vi "LVImplmentation.vi"() -> ()   [LabVIEW 2017]
panel:
  out "Time":dbl
  out "Total":i32
  in  "Multiplier 2":i32
  out "Array 2":i32[](array[numeric])
  out "sum 2":i32
  out "sum":i32
  out "Array":i32[](array[numeric])
  in  "StopThrehold":i32
  in  "Multiplier":i32
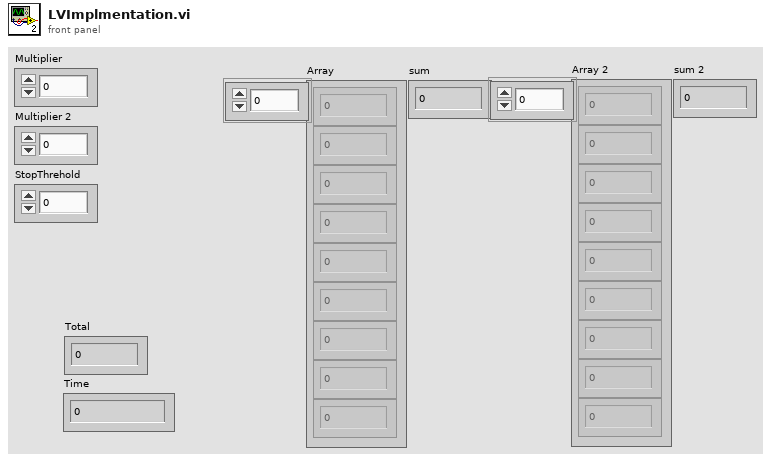
[diagram p1: front panel]
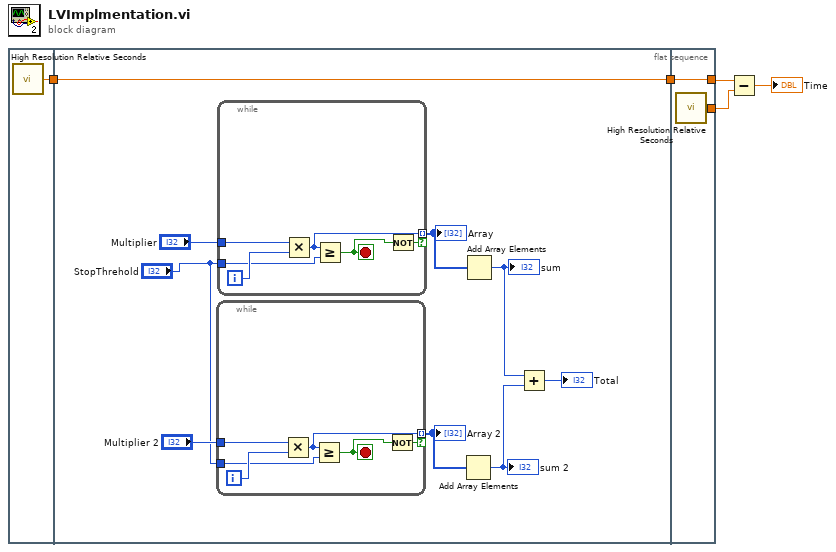
[diagram p0: block diagram]
diagram:
  n1 = flat-sequence {
    tunnel: [w6] -> w4
    tunnel: [w7] -> w5
    tunnel: w4 -> [w7]
    tunnel: [w29] -> w3
    tunnel: w5 -> [w29]
    tunnel: [w28] -> w2
    frame #0 {
      n2 = call <vilib>:"High Resolution Relative Seconds.vi"() -> ("relative seconds"=w6:dbl)
    }
    frame #1 {
      n3 = while {
        tunnel: "Multiplier 2" -> [w20]
        tunnel: "StopThrehold" -> [w19]
        tunnel: [w18] -> w13 mode=indexing if=w16
        i -> [w21]
        stop <- w17 stop-if-true
        n4 = Multiply(x=w20, y=w21) -> (x*y=w18:i32)
        n5 = Greater Or Equal?(x=w18, y=w19) -> (x >= y?=w17:bool)
        n6 = Not(x=w17) -> (.not. x?=w16:bool)
      }
      "Array 2" <- w13
      n7 = while {
        tunnel: "Multiplier" -> [w26]
        tunnel: "StopThrehold" -> [w25]
        tunnel: [w24] -> w14 mode=indexing if=w22
        i -> [w27]
        stop <- w23 stop-if-true
        n8 = Multiply(x=w26, y=w27) -> (x*y=w24:i32)
        n9 = Greater Or Equal?(x=w24, y=w25) -> (x >= y?=w23:bool)
        n10 = Not(x=w23) -> (.not. x?=w22:bool)
      }
      "Array" <- w14
      n11 = Add Array Elements(numeric array=w13) -> (sum=w9:i32)
      "sum 2" <- w9
      n12 = Add Array Elements(numeric array=w14) -> (sum=w10:i32)
      "sum" <- w10
      n13 = Add(x=w10, y=w9) -> (x+y=→"Total":i32)
    }
    frame #2 {
      n14 = call <vilib>:"High Resolution Relative Seconds.vi"() -> ("relative seconds"=w28:dbl)
    }
  }
  n15 = Subtract(x=w3, y=w2) -> (x-y=→"Time":dbl)
